vi "Pick Cell.vi"(1 "# Column":u16, 2 "i Row":i32, 3 "i Column":i32, 7 "Title tous":T1[][](array[typedef])) -> (8 "Cell border":T1)   [LabVIEW 2019]
doc: "Version 1.1\nDeveloped by Jean-Marc Simard\nCopyright © 2012, Exaprom Inc.\nAll rights reserved.\nLicense: BSD\n\nWith iTextSharp 4.1.6 (http://itextsharp.sourceforge.net)\nunder Mozilla Public License Version 1.1\n(http://www.mozilla.org/MPL/MPL-1.1.html)"
uses:
  <userlib>/Exaprom PDF/Controls/Table Controls/Cell Border 20 px.ctl
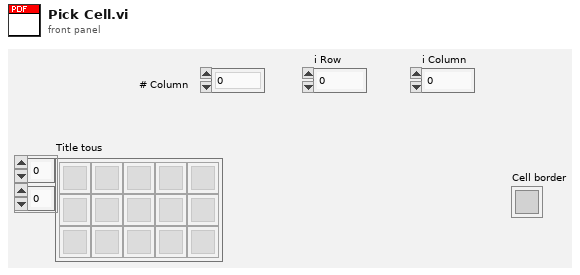
[diagram p1: front panel]
types:
  T1 = typedef "Cell Border 20 px.ctl" = u16
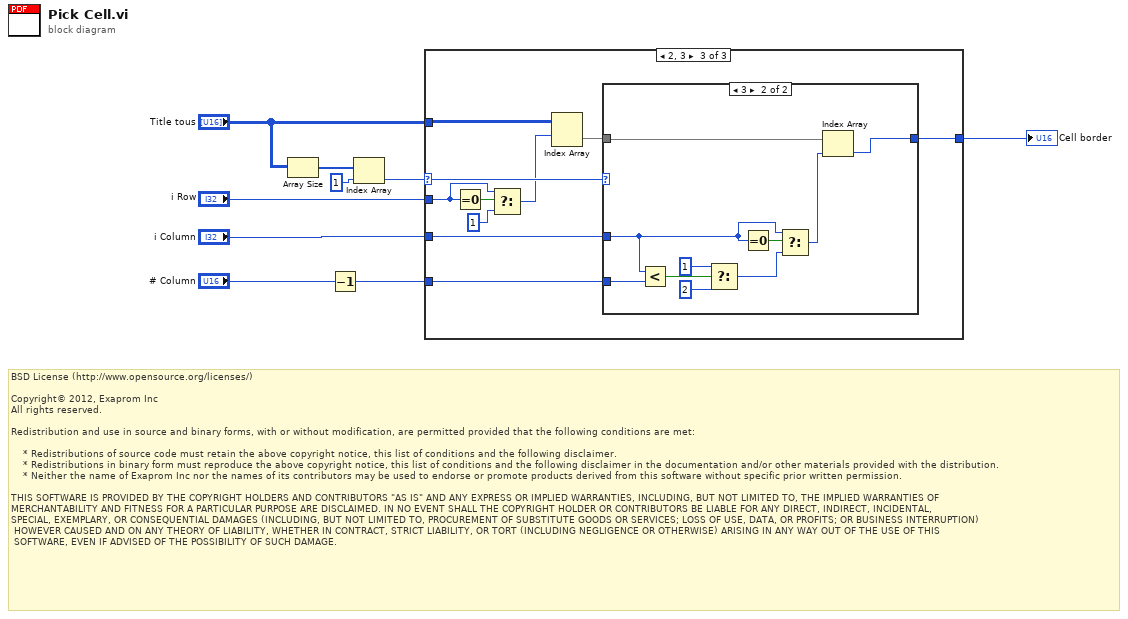
[diagram p0: block diagram]
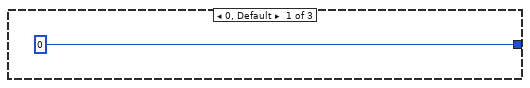
[diagram p2: hidden frame]
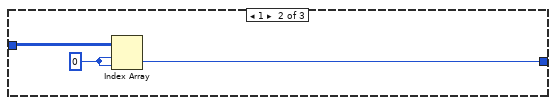
[diagram p3: hidden frame]
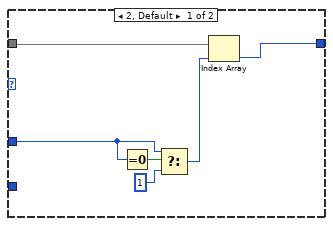
[diagram p4: hidden frame]
diagram:
  # "BSD License (http://www.opensource.org/licenses/)\n\nCopyright© 2012, Exaprom Inc\nAll rights reserved.\n\nRedistribution and use in source and binary forms, with or without modification, are permitted provided that the following conditions are met:\n\n    * Redistributions of source code must retain the above copyright notice, this list of conditions and the following disclaimer.\n    * Redistributions in binary form must reproduce the above copyright notice, this list of conditions and the following disclaimer in the documentation and/or other materials provided with the distribution.\n    * Neither the name of Exaprom Inc nor the names of its contributors may be used to endorse or promote products derived from this software without specific prior written permission.\n\nTHIS SOFTWARE IS PROVIDED BY THE COPYRIGHT HOLDERS AND CONTRIBUTORS \"AS IS\" AND ANY EXPRESS OR IMPLIED WARRANTIES, INCLUDING, BUT NOT LIMITED TO, THE IMPLIED WARRANTIES OF \nMERCHANTABILITY AND FITNESS FOR A PARTICULAR PURPOSE ARE DISCLAIMED. IN NO EVENT SHALL THE COPYRIGHT HOLDER OR CONTRIBUTORS BE LIABLE FOR ANY DIRECT, INDIRECT, INCIDENTAL,\nSPECIAL, EXEMPLARY, OR CONSEQUENTIAL DAMAGES (INCLUDING, BUT NOT LIMITED TO, PROCUREMENT OF SUBSTITUTE GOODS OR SERVICES; LOSS OF USE, DATA, OR PROFITS; OR BUSINESS INTERRUPTION)\n HOWEVER CAUSED AND ON ANY THEORY OF LIABILITY, WHETHER IN CONTRACT, STRICT LIABILITY, OR TORT (INCLUDING NEGLIGENCE OR OTHERWISE) ARISING IN ANY WAY OUT OF THE USE OF THIS\n SOFTWARE, EVEN IF ADVISED OF THE POSSIBILITY OF SUCH DAMAGE."
  n1 = Array Size(array="Title tous") -> (size(s)=w9:i32[])
  n2 = Decrement(x="# Column") -> (x-1=w1:u16)
  n3 = Index Array(array=w9, index=1) -> (element=w7:i32)
  n4 = case shown="2, 3" w7 {
    selector: w7 -> [_ _ w20]
    tunnel: "Title tous" -> [_ w13 w23]
    tunnel: [T1 0 ("Cell border") w11 w16] -> w5
    tunnel: "i Row" -> [_ _ w19]
    tunnel: "i Column" -> [_ _ w15]
    tunnel: w1 -> [_ _ w18]
    frame 0, Default {
    }
    frame 1 {
      w12 = 0 ("index (row)")
      n5 = Index Array(array=w13, index (row)=w12, index (col)=w12) -> (element=w11:T1)
    }
    frame 2, 3 {
      n6 = Equal To 0?(x=w19) -> (x = 0?=w22:bool)
      n7 = Select(t=w19, s=w22, f=1 ("disabled index (col)")) -> (s? t:f=w14:i32)
      n8 = Index Array(array=w23, index (row)=w14) -> (element=w17:T1[])  [unwired: 1 in]
      n9 = case shown="3" w20 {
        tunnel: w15 -> [w25 w35]
        tunnel: w18 -> [_ w34]
        tunnel: w17 -> [w29 w39]
        tunnel: [w28 w38] -> w16
        frame 2, Default {
          n10 = Equal To 0?(x=w25) -> (x = 0?=w26:bool)
          n11 = Select(t=w25, s=w26, f=1 ("disabled index (col)")) -> (s? t:f=w24:i32)
          n12 = Index Array(array=w29, index=w24) -> (element=w28:T1)
        }
        frame 3 {
          n13 = Less?(x=w35, y=w34) -> (x < y?=w33:bool)
          n14 = Select(t=u16 1, s=w33, f=u16 2) -> (s? t:f=w32:u16)
          n15 = Equal To 0?(x=w35) -> (x = 0?=w37:bool)
          n16 = Select(t=w35, s=w37, f=w32) -> (s? t:f=w36:i32)
          n17 = Index Array(array=w39, index=w36) -> (element=w38:T1)
        }
      }
    }
  }
  "Cell border" <- w5
